vi "Do.vi"(8 "error in (no error)":errorcluster, 10 "DMM":refnum<class "DMM.lvclass">, 11 "Initialize in":refnum<class "Initialize.lvclass">) -> (0 "error out":errorcluster, 2 "DMM":refnum<class "DMM.lvclass">, 3 "Initialize out":refnum<class "Initialize.lvclass">)   [LabVIEW 2020, in "Initialize.lvclass"]
uses:
  Initialize.lvclass
  DMM/DMM.lvclass
  Initialize.lvclass/Initialize.ctl
  DMM/DMM.lvclass/DMM.ctl
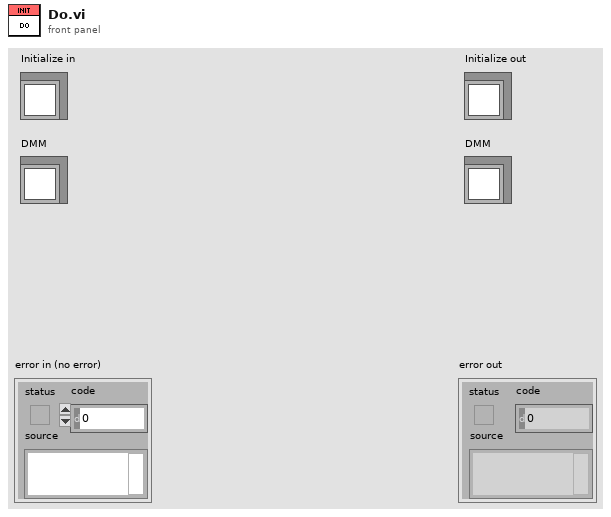
[diagram p1: front panel]
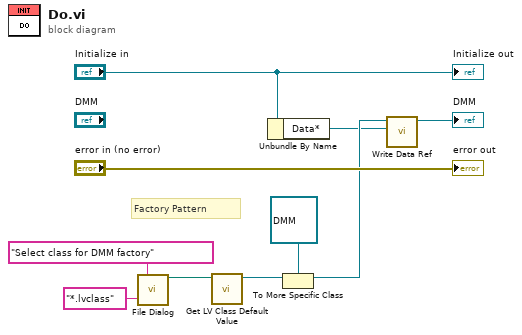
[diagram p0: block diagram]
diagram:
  # "Factory Pattern"
  n1 = call "File Dialog"("prompt"="Select class for DMM factory", "pattern (all files)"="*.lvclass") -> ("selected path"=w6:path)  [unwired: 10 in, 3 out]
  n2 = call <vilib>:"Get LV Class Default Value.vi"("class path"=w6) -> ("object"=w9:refnum<class>)  [unwired: 9 in, 1 out]
  n3 = Unbundle By Name("Initialize in") -> ("Data*"=w1:refnum<vi>)
  n4 = To More Specific Class(target class=refnum<class "DMM.lvclass"> refnum ("DMM.lvclass"), reference=w9) -> (specific class reference=w3:refnum<class "DMM.lvclass">)  [unwired: 1 in, 1 out]
  n5 = call "Write Data Ref.vi"("Data*"=w1, "DMM in"=w3) -> ("DMM out"=→"DMM":refnum<class "DMM.lvclass">)  [unwired: 8 in, 1 out]
  "error out" <- "error in (no error)"
  "Initialize out" <- "Initialize in"
